vi "Write columns.vi"(8 "error in (no error)":errorcluster, 10 "columns":string[](array[string]), 11 "DbMeasurement in":refnum<class "DbMeasurement.lvclass">) -> (0 "error out":errorcluster, 3 "DbMeasurement out":refnum<class "DbMeasurement.lvclass">)   [LabVIEW 2013, in "DbMeasurement.lvclass"]
doc: "This accessor sets the column name array used to specify data columns in the database."
uses:
  DbMeasurement.lvclass
  DbMeasurement.lvclass/DbMeasurement.ctl
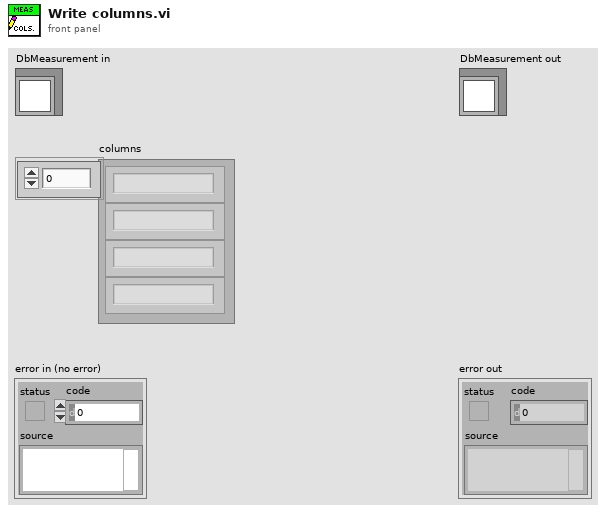
[diagram p1: front panel]
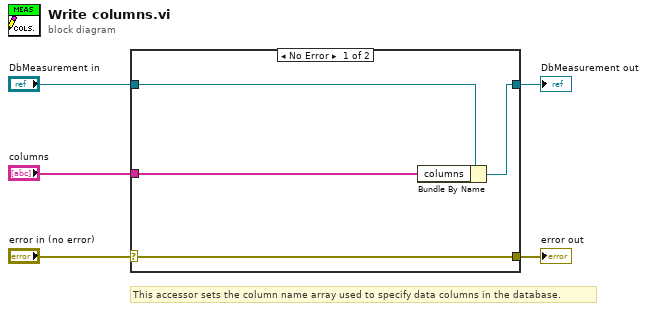
[diagram p0: block diagram]
diagram:
  # "This accessor sets the column name array used to specify data columns in the database."
  n1 = case shown="No Error" "error in (no error)" {
    selector: "error in (no error)" -> [w9 w10]
    tunnel: [w9 w10] -> w4
    tunnel: [w7 w11] -> w2
    tunnel: "DbMeasurement in" -> [w8 w11]
    tunnel: "columns" -> [w6 _]
    frame No Error {
      n2 = Bundle By Name(cluster=w8, "columns"=w6) -> (w7:refnum<class "DbMeasurement.lvclass">)
    }
    frame Error {
    }
  }
  "error out" <- w4
  "DbMeasurement out" <- w2
